vi "VSSDetectionFIRASimField.vi"(8 "error in (no error)":errorcluster, 11 "Field":u8[](array[numeric]) format="%02x") -> (0 "error out":errorcluster, 2 "Goals":u8[](array[numeric]), 3 "Field out":T1)   [LabVIEW 2023]
panel:
  in  "Field":T1
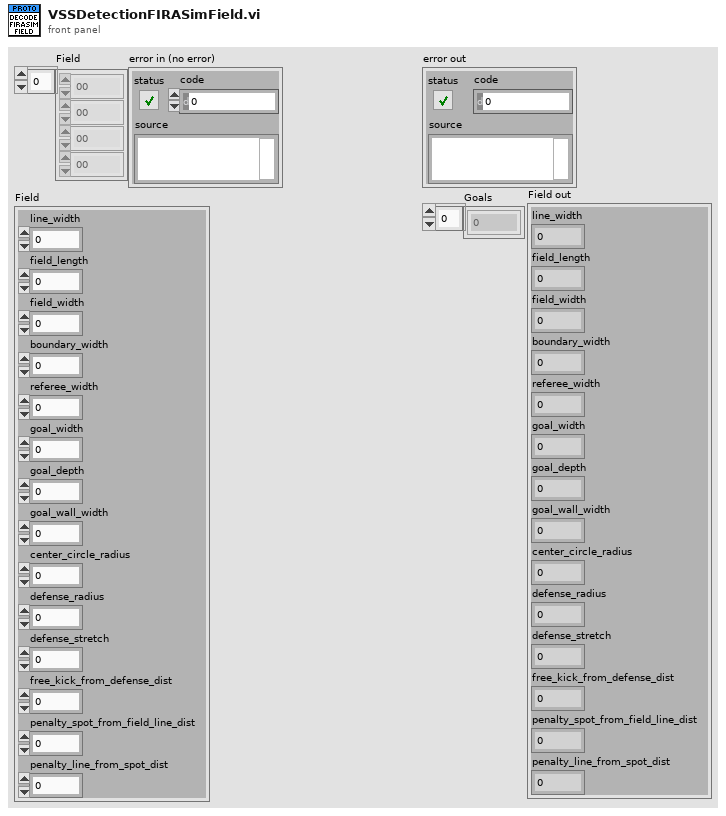
[diagram p1: front panel]
types:
  T1 = cluster{"line_width":u32, "field_length":u32, "field_width":u32, "boundary_width":u32, "referee_width":u32, "goal_width":u32, "goal_depth":u32, "goal_wall_width":u32, "center_circle_radius":u32, "defense_radius":u32, "defense_stretch":u32, "free_kick_from_defense_dist":u32, "penalty_spot_from_field_line_dist":u32, "penalty_line_from_spot_dist":u32}
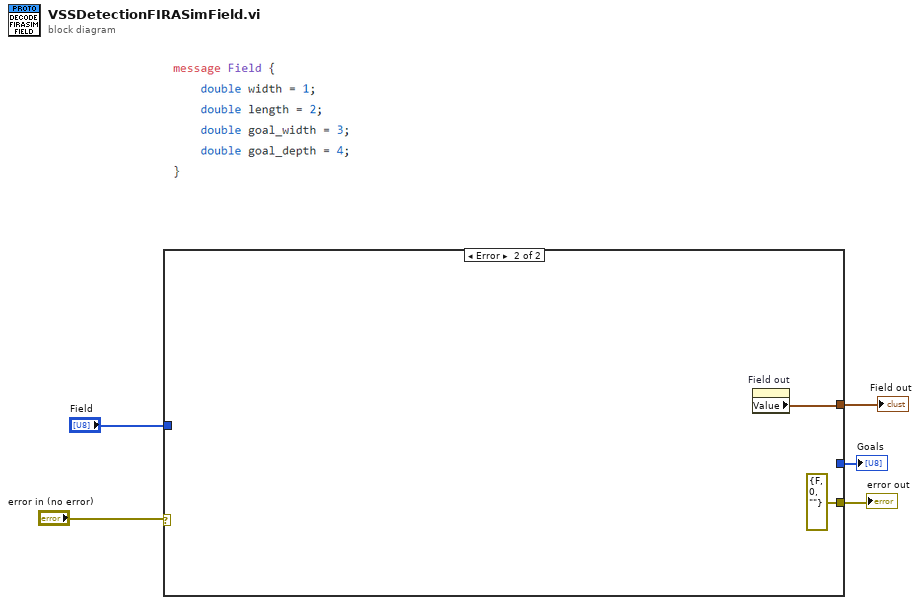
[diagram p0: block diagram]
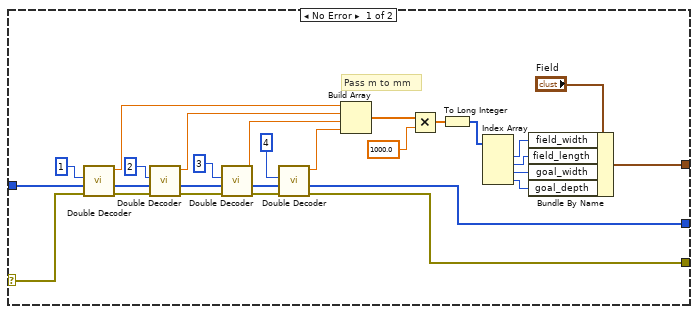
[diagram p2: hidden frame]
diagram:
  n1 = case shown="Error" "error in (no error)" {
    selector: "error in (no error)" -> [w30 _]
    tunnel: "Field" -> [w32 _]
    tunnel: [w8 _] -> w3
    tunnel: [w7 w35] -> w2
    tunnel: [w6 errorcluster {"status"=FALSE, "code"=0, "source"=""} ("error out")] -> w1
    frame No Error {
      # "Pass m to mm"
      n2 = call "Double Decoder.vi"("error in (no error)"=w30, "Array"=w32, "Key"=1) -> ("error out"=w29:errorcluster, "array w/ subset deleted"=w28:u8[], "Double"=w20:dbl)  [unwired: 5 in, 1 out]
      n3 = call "Double Decoder.vi"("error in (no error)"=w29, "Array"=w28, "Key"=2) -> ("error out"=w26:errorcluster, "array w/ subset deleted"=w24:u8[], "Double"=w19:dbl)  [unwired: 5 in, 1 out]
      n4 = call "Double Decoder.vi"("error in (no error)"=w26, "Array"=w24, "Key"=3) -> ("error out"=w25:errorcluster, "array w/ subset deleted"=w23:u8[], "Double"=w18:dbl)  [unwired: 5 in, 1 out]
      n5 = call "Double Decoder.vi"("error in (no error)"=w25, "Array"=w23, "Key"=4) -> ("error out"=w6:errorcluster, "array w/ subset deleted"=w8:u8[], "Double"=w17:dbl)  [unwired: 5 in, 1 out]
      n6 = Build Array(w20, w19, w18, w17) -> (w16:dbl[])
      n7 = Multiply(x=w16, y=1000.0) -> (x*y=w14:dbl[])
      n8 = To Long Integer(number=w14) -> (32bit integer=w13:i32[])
      n9 = Index Array(array=w13) -> (element #1=w12:i32, element #2=w11:i32, element #3=w10:i32, element #4=w9:i32)  [unwired: 4 in]
      n10 = Bundle By Name(cluster="Field", "field_width"=w12, "field_length"=w11, "goal_width"=w10, "goal_depth"=w9) -> (w7:T1)
    }
    frame Error {
      n11 = property on="Field out" class="Clust (strict)"() -> ("Value"=w35:T1)  [unwired: 2 in, 2 out]
    }
  }
  "error out" <- w1
  "Goals" <- w3
  "Field out" <- w2
